vi "Update SubPanel.vi"(8 "error in (no error)":errorcluster, 11 "Manager in":refnum<class "Manager.lvclass">) -> (0 "error out":errorcluster, 3 "Manager out":refnum<class "Manager.lvclass">)   [LabVIEW 2012, in "Manager.lvlib" / "Manager.lvclass"]
uses:
  Manager.lvclass
  Manager.lvclass/Manager.ctl
  Bioreactor Actor/Bioreactor Messages/View Front Panel Msg/View Front Panel Msg.lvclass/View Front Panel Msg.ctl
  <vilib>/ActorFramework/Message Enqueuer/Message Enqueuer.lvclass/Message Enqueuer.ctl
  Time Protocol Actor/Time Protocol Messages/View Front Panel Msg/View Front Panel Msg.lvclass/View Front Panel Msg.ctl
  Python Protocol Actor/Python Protocol Messages/View Front Panel Msg/View Front Panel Msg.lvclass/View Front Panel Msg.ctl
  Read Control Systems.vi
  Read System Ring Refnum.vi
  Read Actor Ring Refnum.vi
  Read SubPnl Refnum.vi
  <vilib>/ActorFramework/Message Enqueuer/Enqueue.vi
  <vilib>/ActorFramework/Message Priority Queue/Priority Enqueue.vi
  <vilib>/ActorFramework/Message Enqueuer/Message Enqueuer.lvclass
  Bioreactor Actor/Bioreactor Messages/View Front Panel Msg/View Front Panel Msg.lvclass
  Time Protocol Actor/Time Protocol Messages/View Front Panel Msg/View Front Panel Msg.lvclass
  Python Protocol Actor/Python Protocol Messages/View Front Panel Msg/View Front Panel Msg.lvclass
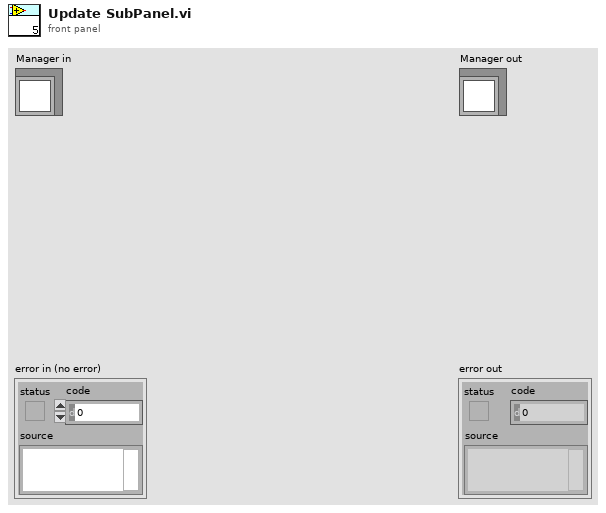
[diagram p1: front panel]
types:
  T1 = cluster{"Bioreactor Queue":refnum<class "Message Enqueuer.lvclass">, "Time Protocol Queue":refnum<class "Message Enqueuer.lvclass">, "Python Protocol Queue":refnum<class "Message Enqueuer.lvclass">, "Name":string}[]
  T2 = cluster{"Bioreactor Queue":refnum<class "Message Enqueuer.lvclass">, "Time Protocol Queue":refnum<class "Message Enqueuer.lvclass">, "Python Protocol Queue":refnum<class "Message Enqueuer.lvclass">, "Name":string}
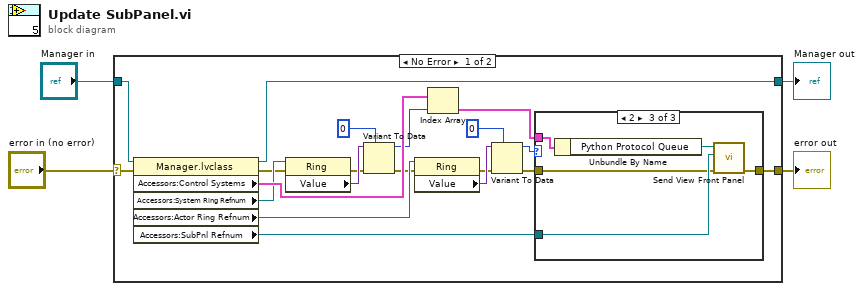
[diagram p0: block diagram]
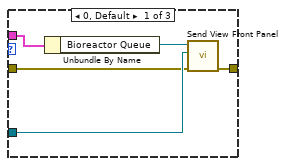
[diagram p2: hidden frame]
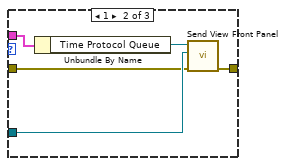
[diagram p3: hidden frame]
diagram:
  n1 = case shown="No Error" "error in (no error)" {
    selector: "error in (no error)" -> [w11 w41]
    tunnel: [w5 w41] -> w3
    tunnel: [w12 w40] -> w1
    tunnel: "Manager in" -> [w24 w40]
    frame No Error {
      n2 = property class="Manager.lvclass"(reference=w24, error in=w11) -> (reference out=w12:refnum<class "Manager.lvclass">, error out=w10:errorcluster, "Accessors:Control Systems"=w23:T1, "Accessors:System Ring Refnum"=w22:refnum<vi>, "Accessors:Actor Ring Refnum"=w16:refnum<vi>, "Accessors:SubPnl Refnum"=w13:refnum<vi>)
      n3 = property class="Ring"(reference=w22, error in=w10) -> (error out=w9:errorcluster, "Value"=w20:variant)  [unwired: 1 out]
      n4 = Variant To Data(error in=w9, type=0, Variant=w20) -> (data=w19:i32, error out=w8:errorcluster)
      n5 = property class="Ring"(reference=w16, error in=w8) -> (error out=w7:errorcluster, "Value"=w17:variant)  [unwired: 1 out]
      n6 = Index Array(array=w23, index=w19) -> (element=w14:T2)
      n7 = Variant To Data(error in=w7, type=0, Variant=w17) -> (data=w15:i32, error out=w6:errorcluster)
      n8 = case shown="2" w15 {
        tunnel: w14 -> [w29 w34 w39]
        tunnel: w13 -> [w27 w32 w37]
        tunnel: w6 -> [w26 w31 w36]
        tunnel: [w25 w30 w35] -> w5
        frame 0, Default {
          n9 = Unbundle By Name(w29) -> ("Bioreactor Queue"=w28:refnum<class "Message Enqueuer.lvclass">)
          n10 = call "Send View Front Panel.vi"("error in (no error)"=w26, "SubPnl Refnum"=w27, "Message Enqueuer"=w28) -> ("error out"=w25:errorcluster)  [unwired: 7 in, 1 out]
        }
        frame 1 {
          n11 = Unbundle By Name(w34) -> ("Time Protocol Queue"=w33:refnum<class "Message Enqueuer.lvclass">)
          n12 = call "Send View Front Panel.vi"("error in (no error)"=w31, "SubPnl Refnum"=w32, "Message Enqueuer"=w33) -> ("error out"=w30:errorcluster)  [unwired: 7 in, 1 out]
        }
        frame 2 {
          n13 = Unbundle By Name(w39) -> ("Python Protocol Queue"=w38:refnum<class "Message Enqueuer.lvclass">)
          n14 = call "Send View Front Panel.vi"("error in (no error)"=w36, "SubPnl Refnum"=w37, "Message Enqueuer"=w38) -> ("error out"=w35:errorcluster)  [unwired: 7 in, 1 out]
        }
      }
    }
    frame Error {
    }
  }
  "error out" <- w3
  "Manager out" <- w1
